vi "Write New Data Msg.vi"(10 "Nested Actor.lvlib:New Data Msg.lvclass":refnum<class "New Data Msg.lvclass">, 11 "Nested Actor in":refnum<class "Nested Actor.lvclass">) -> (3 "Nested Actor out":refnum<class "Nested Actor.lvclass">)   [LabVIEW 2018, in "Nested Actor.lvlib" / "Nested Actor.lvclass"]
uses:
  Nested Actor.lvclass
  Nested Actor Messages/New Data Msg/New Data Msg.lvclass
  Nested Actor.lvclass/Nested Actor.ctl
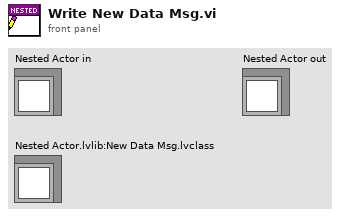
[diagram p1: front panel]
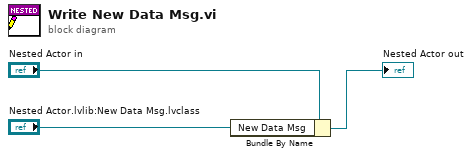
[diagram p0: block diagram]
diagram:
  n1 = Bundle By Name(cluster="Nested Actor in", "New Data Msg"="Nested Actor.lvlib:New Data Msg.lvclass") -> (→"Nested Actor out":refnum<class "Nested Actor.lvclass">)
